vi "JsonToCluster.vi"(11 "Response body":string) -> (3 "Cluster":T1)   [LabVIEW 2020]
uses:
  <vilib>/addons/_JKI.lib/Serialization/JSON/JKI JSON Serialization.lvlib
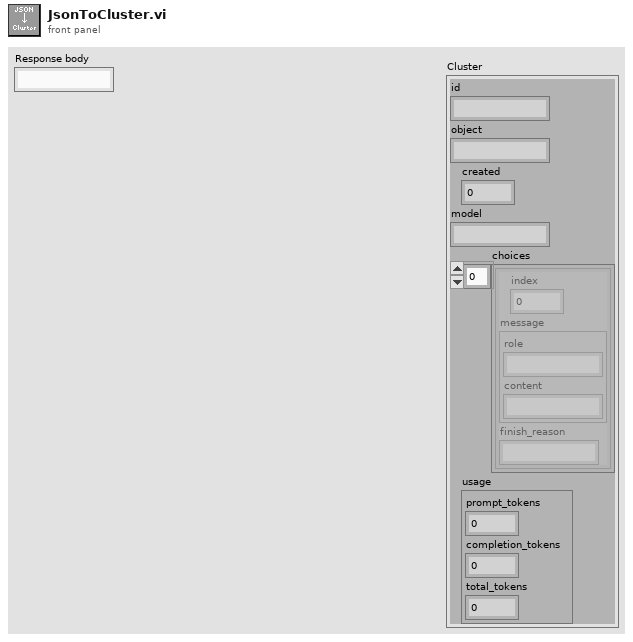
[diagram p1: front panel]
types:
  T1 = cluster{"id":string, "object":string, "created":i32, "model":string, "choices":cluster{"index":i32, "message":cluster{"role":string, "content":string}, "finish_reason":string}[], "usage":cluster{"prompt_tokens":i32, "completion_tokens":i32, "total_tokens":i32}}
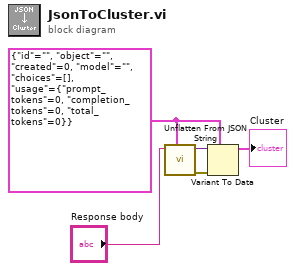
[diagram p0: block diagram]
diagram:
  w4 = T1 {"id"="", "object"="", "created"=0, "model"="", "choices"=[], "usage"={"prompt_tokens"=0, "completion_tokens"=0, "total_tokens"=0}}
  n1 = call <vilib>:"Unflatten From JSON String.vi"("Type and Defaults"=w4, "JSON String"="Response body") -> ("error out"=w2:errorcluster, "Variant"=w3:variant)  [unwired: 8 in]
  n2 = Variant To Data(error in=w2, type=w4, Variant=w3) -> (data=→"Cluster":T1)  [unwired: 1 out]
